vi "3_2_Señales.vi"(0 "Offset":dbl(knob) scale=0.0..10.0, 2 "Reset Signal":bool, 5 "Frecuencia (Hz)":dbl(knob)=10.1 caption="Frequency" scale=0.0..500.0 scale format="%#.6g", 7 "Amplitud (V)":dbl(knob)=1.0 caption="Amplitude" scale=0.0..10.0 scale format="%#.1g", 9 "Fase (°)":dbl(knob) caption="Phase" step=1.0 scale=-90.0..90.0, 11 "error in (no error)":errorcluster) -> (4 "Señales":dynamicdata(graph) caption="Sine", 15 "error out":errorcluster)   [LabVIEW 2020]
doc: "Simulates a sine wave, square wave, triangle wave, sawtooth wave, or noise signal.\n--------------------\n\nThis Express VI is configured as follows:\n\nSignal Type: Sine\nFrequency: 10.1 Hz\nAmplitude: 1\nPhase: 0\nOffset: 0\nSampling Rate: 1000 Hz\nNumber of Samples: 100 (Automatic)\nTiming: Run as fast as possible\nTimestamps: Relative"
panel:
  in  "Ruido 2":bool
  in  "Tipo de Ruido 2":u16(ring) items=["Uniform White Noise", "Gaussian White Noise", "Periodic Random Noise", "Gamma Noise", "Poisson Noise", "Binomial Noise", "Bernoulli Noise", "MLS Sequence "]
  in  "TIPO DE SEÑAL 2":u16(ring) items=["Sine", "Square", "Triangle", "Sawtooth", "DC"]
  in  "Trials 2":i32=1 caption="Trials"
  in  "Seed Number 2":dbl=-1.0 caption="Seed Number"
  in  "Amplitud de Ruido (V) 2":dbl(slide)=0.6 caption="Noise amplitude" step=0.1 scale=0.0..10.0
  out "error out 2":errorcluster caption="error out"
  in  "Reset Signal 2":bool caption="Reset Signal"
  in  "error in (no error) 2":errorcluster caption="error in (no error)"
  in  "Ciclo de Trabajo (%) 2":dbl(knob)=50.0 caption="Duty Cycle (%)" scale=0.0..100.0
  in  "Fase (°) 2":dbl(knob) caption="Phase" step=1.0 scale=-90.0..90.0
  in  "Amplitud (V) 2":dbl(knob)=1.0 caption="Amplitude" scale=0.0..10.0 scale format="%#.1g"
  in  "Frecuencia (Hz) 2":dbl(knob)=10.1 caption="Frequency" scale=0.0..500.0 scale format="%#.6g"
  in  "Offset 2":dbl(knob) caption="Offset" scale=0.0..20.0
  in  "Ruido":bool
  in  "Tipo de Ruido":u16(ring) items=["Uniform White Noise", "Gaussian White Noise", "Periodic Random Noise", "Gamma Noise", "Poisson Noise", "Binomial Noise", "Bernoulli Noise", "MLS Sequence "]
  in  "TIPO DE SEÑAL":u16(ring) items=["Sine", "Square", "Triangle", "Sawtooth", "DC"]
  in  "?":bool
  in  "Trials":i32=1
  in  "Seed Number":dbl=-1.0
  in  "Amplitud de Ruido (V)":dbl(slide)=0.6 caption="Noise amplitude" step=0.1 scale=0.0..10.0
  in  "Ciclo de Trabajo (%)":dbl(knob)=50.0 caption="Duty Cycle (%)" scale=0.0..100.0
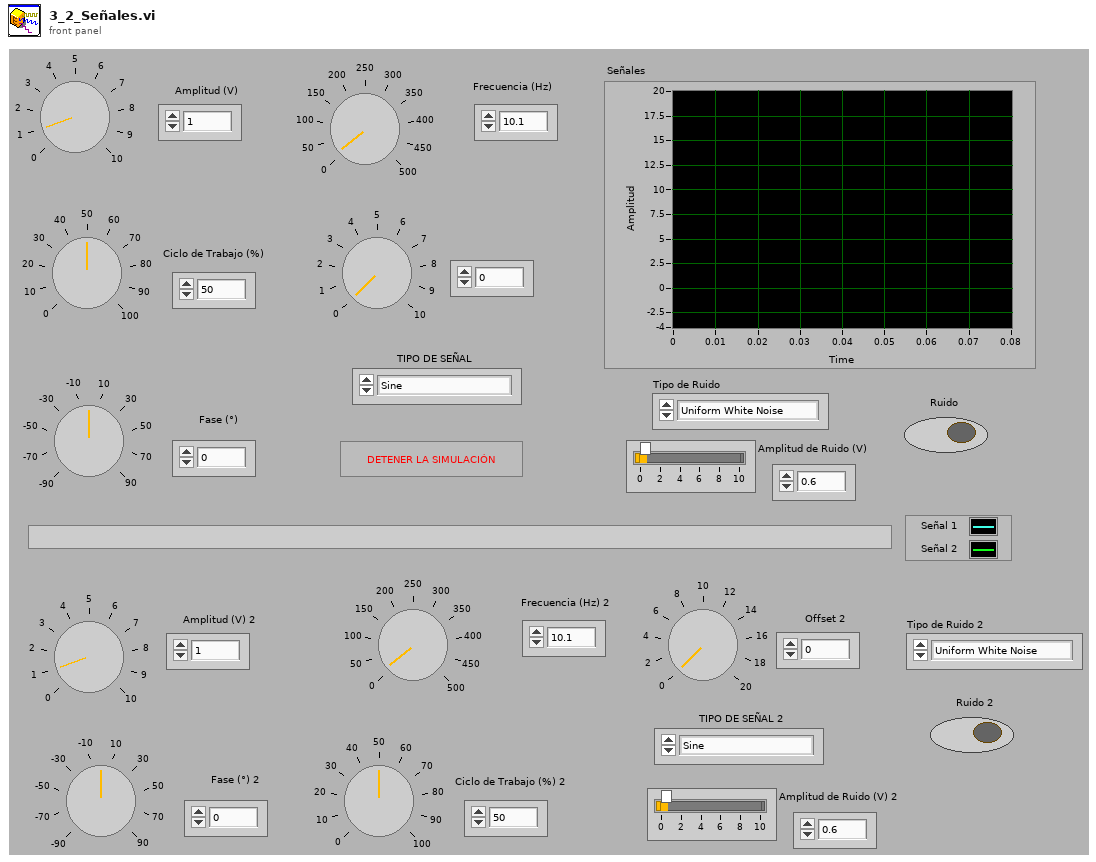
[diagram p1: front panel]
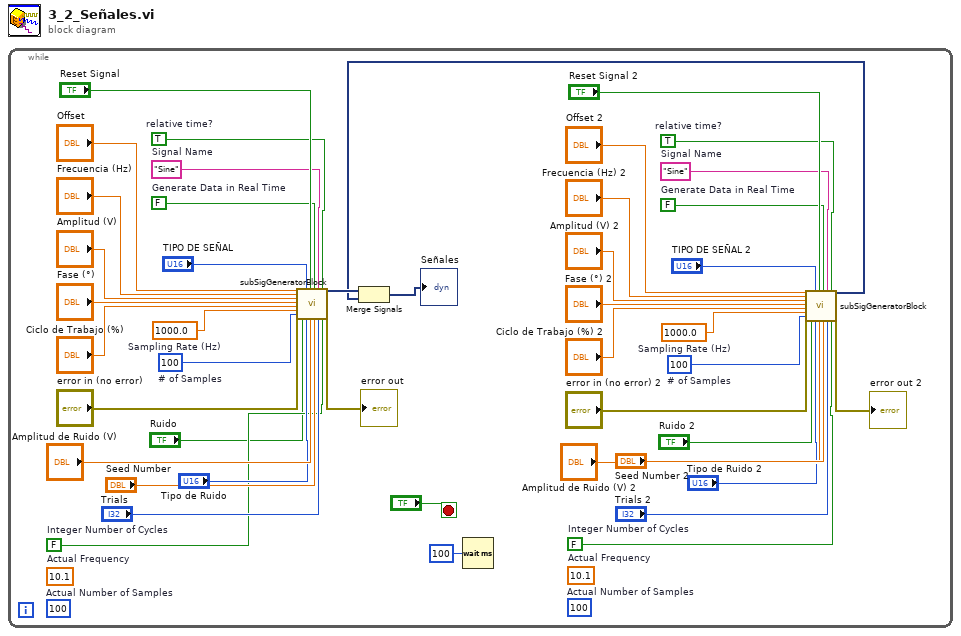
[diagram p0: block diagram]
diagram:
  n1 = while {
    stop <- "?" stop-if-true
    (unwired) 10.1  # Actual Frequency
    (unwired) 100  # Actual Number of Samples
    w5 = FALSE  # Integer Number of Cycles
    w6 = TRUE  # relative time?
    w7 = "Sine"  # Signal Name
    w8 = FALSE  # Generate Data in Real Time
    w11 = 100  # # of Samples
    w12 = 1000.0  # Sampling Rate (Hz)
    (unwired) 10.1  # Actual Frequency
    (unwired) 100  # Actual Number of Samples
    w26 = FALSE  # Integer Number of Cycles
    w27 = TRUE  # relative time?
    w28 = "Sine"  # Signal Name
    w29 = FALSE  # Generate Data in Real Time
    w32 = 100  # # of Samples
    w33 = 1000.0  # Sampling Rate (Hz)
    n2 = call <vilib>:"subSigGeneratorBlock.vi"("Offset"="Offset", "Frequency"="Frecuencia (Hz)", "Amplitude"="Amplitud (V)", "Phase"="Fase (°)", "Duty Cycle (%)"="Ciclo de Trabajo (%)", "Sampling Rate (Hz)"=w33, "# of Samples"=w32, "error in (no error)"="error in (no error)", "Noise"="Ruido", "Generate"="TIPO DE SEÑAL", "Noise Ring"="Tipo de Ruido", "Reset Signal"="Reset Signal", "Noise Amplitude"="Amplitud de Ruido (V)", "Generate Data in Real Time"=w29, "Seed Number"="Seed Number", "Signal Name"=w28, "trials"="Trials", "relative time?"=w27, "Integer Number of Cycles"=w26) -> ("Signal"=w41:dynamicdata, "error out"=→"error out":errorcluster)  [unwired: 7 in]
    n3 = Wait (ms)(milliseconds to wait=u32 100) -> ()  [unwired: 1 out]
    n4 = call <vilib>:"subSigGeneratorBlock.vi"("Offset"="Offset 2", "Frequency"="Frecuencia (Hz) 2", "Amplitude"="Amplitud (V) 2", "Phase"="Fase (°) 2", "Duty Cycle (%)"="Ciclo de Trabajo (%) 2", "Sampling Rate (Hz)"=w12, "# of Samples"=w11, "error in (no error)"="error in (no error) 2", "Noise"="Ruido 2", "Generate"="TIPO DE SEÑAL 2", "Noise Ring"="Tipo de Ruido 2", "Reset Signal"="Reset Signal 2", "Noise Amplitude"="Amplitud de Ruido (V) 2", "Generate Data in Real Time"=w8, "Seed Number"="Seed Number 2", "Signal Name"=w7, "trials"="Trials 2", "relative time?"=w6, "Integer Number of Cycles"=w5) -> ("Signal"=w2:dynamicdata, "error out"=→"error out 2":errorcluster)  [unwired: 7 in]
    n5 = Merge Signals(w41, w2) -> (→"Señales":dynamicdata)
  }
